vi "Set Point.vi"(8 "error in (no error)":errorcluster, 10 "Set point":dbl, 11 "Neocera Driver in":refnum<class "Neocera Driver.lvclass">) -> (0 "error out":errorcluster, 3 "Neocera Driver out":refnum<class "Neocera Driver.lvclass">)   [LabVIEW 2016, in "Neocera Driver.lvclass"]
uses:
  Neocera Driver.lvclass
  C:/github/NHMFL_Core/Libraries/Instruments/VISA Instrument/VISA Instrument.lvclass
  VISA Instrument/VISA Instrument.lvclass/VISA Instrument.ctl
  VISA Instrument/Read VISA resource.vi
  VISA Instrument/Write VISA resource.vi
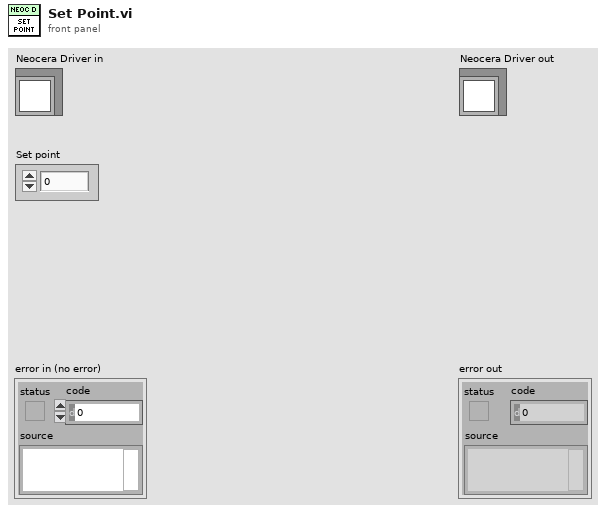
[diagram p1: front panel]
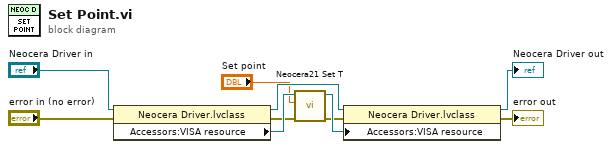
[diagram p0: block diagram]
diagram:
  n1 = property class="Neocera Driver.lvclass"(reference="Neocera Driver in", error in="error in (no error)") -> (reference out=w10:refnum<class "Neocera Driver.lvclass">, error out=w2:errorcluster, "Accessors:VISA resource"=w5:refnum<visa-resource-name>)
  n2 = call "Neocera21 Set T.vi"("error in (no error)"=w2, "Set T"="Set point", "VISA Resource Name"=w5) -> ("error out"=w3:errorcluster, "VISA Resource Name Out"=w4:refnum<visa-resource-name>)  [unwired: 7 in]
  n3 = property class="Neocera Driver.lvclass"(reference=w10, error in=w3, "Accessors:VISA resource"=w4) -> (reference out=→"Neocera Driver out":refnum<class "Neocera Driver.lvclass">, error out=→"error out":errorcluster)
